vi "ASIC_CONFIGURAR DAC MUX.vi"(7 "Espera acceso USB":u32=10, 8 "error in":errorcluster, 10 "dac mux(0..7)":T1, 11 "ftHandle_in":u32) -> (0 "error out":errorcluster, 1 "Write OK":bool, 3 "ftHandle_out":u32)   [LabVIEW 2019]
uses:
  ASIC_Valores dac_mux_ena.ctl
panel:
  out "test":u16 format="%04x"
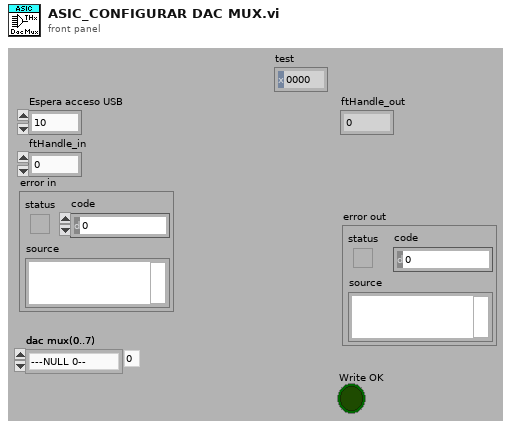
[diagram p1: front panel]
types:
  T1 = typedef "ASIC_Valores dac_mux_ena.ctl" = enum16{"---NULL 0--", "HLTH0 (ADD A)", "HLTH1 (ADD B)", "HLTH2 (ADD C)", "LLTH0 (ADD A)", "LLTH1 (ADD B)", "LLTH2 (ADD C)", "---NULL 1--"}
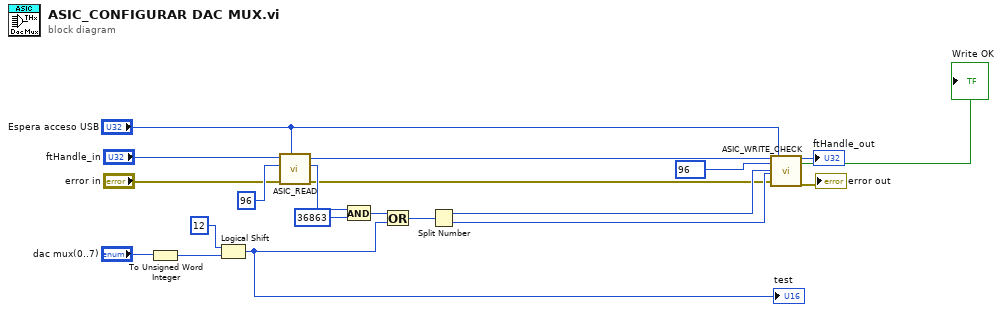
[diagram p0: block diagram]
diagram:
  n1 = To Unsigned Word Integer(number="dac mux(0..7)") -> (unsigned 16bit integer=w3:u16)
  n2 = Logical Shift(y=u16 12 ("x"), x=w3) -> (x << y=w6:u16)
  "test" <- w6
  n3 = call "ASIC_READ.vi"("Espera acceso USB"="Espera acceso USB", "error in"="error in", "Direccion Registro Asic"=u8 96, "ftHandle_in"="ftHandle_in") -> ("error out"=w2:errorcluster, "Valor Asic"=w9:u16, "ftHandle_out"=w12:u32)  [unwired: 5 in]
  n4 = And(x=w9, y=u16 36863) -> (x .and. y?=w7:u16)
  n5 = Or(x=w7, y=w6) -> (x .or. y?=w5:u16)
  n6 = Split Number(x=w5) -> (hi(x)=w11:u8, lo(x)=w10:u8)
  n7 = call "ASIC_WRITE_CHECK.vi"("ftHandle_in"=w12, "Direccion Registro Asic"=u8 96, "Byte Alto"=w11, "Byte Bajo"=w10, "error in"=w2, "Espera acceso USB 2"="Espera acceso USB") -> ("ftHandle_out"=→"ftHandle_out":u32, "Write OK"=→"Write OK":bool, "error out"=→"error out":errorcluster)  [unwired: 11 in]
